vi "check_for_parse_errors.vi"(6 "just check details? (false: also raise labview error)":bool, 7 "optional file path (to include in parse error message)":path, 8 "error in (no error)":errorcluster, 11 "toml":string) -> (0 "error out":errorcluster, 1 "error details":string, 2 "error occurred?":bool)   [LabVIEW 2020, in "toml_edit.lvlib" / "Doc.lvclass"]
uses:
  Doc.lvclass
  <userlib>/_OpenG.lib/file/file.llb/Valid Path - Traditional__ogtk.vi
  toml_edit.lvlib
  <userlib>/_OpenG.lib/file/file.llb/openg_file.lvlib
  dragon_toml_64.dll
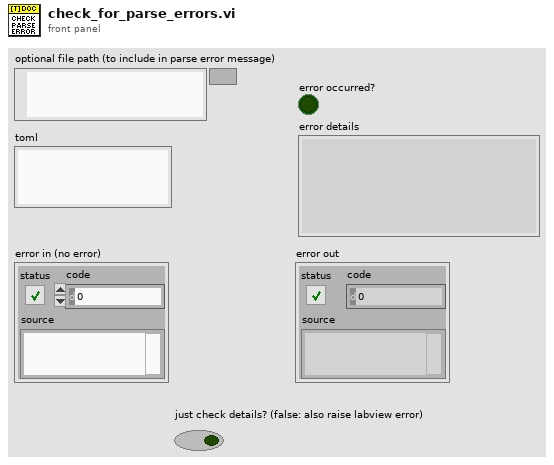
[diagram p1: front panel]
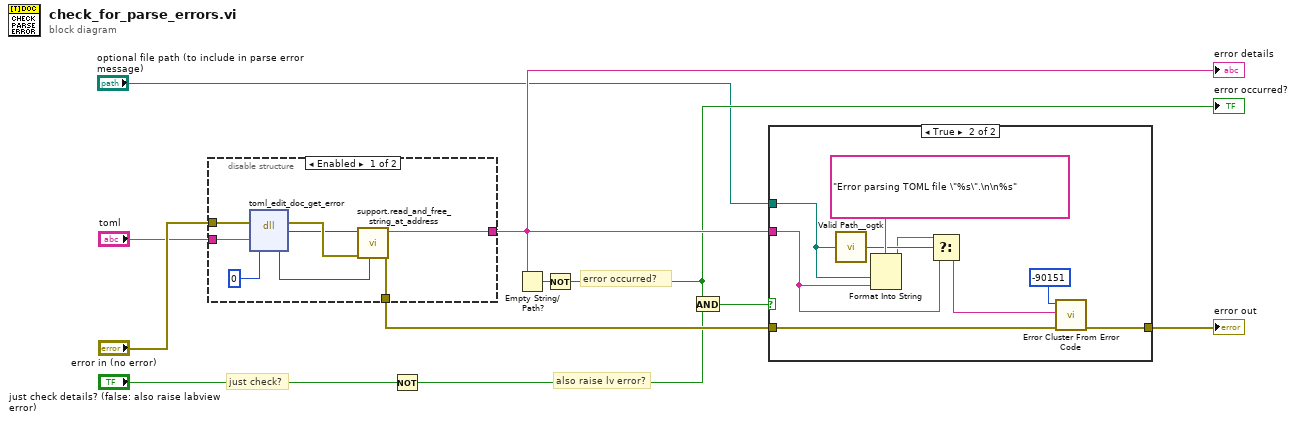
[diagram p0: block diagram]
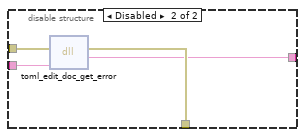
[diagram p2: hidden frame]
diagram:
  # "error occurred?"
  # "just check?"
  # "also raise lv error?"
  n1 = disable-structure shown="Enabled" {
    disable-tunnel: [w19 w21] -> w11
    disable-tunnel: [w18 w23] -> w8
    disable-tunnel: "error in (no error)" -> [w16 w22]
    disable-tunnel: "toml" -> [w14 w20]
    frame Enabled {
      n2 = dll-call lib="C:/projects/dragon-desktop/source/submodules/toml-edit-labview/lv_src/dragon_toml_*.*" fn="toml_edit_doc_get_error"(error in=w16, "toml_string"=w14, "string_length"=u32 0) -> (error out=w17:errorcluster, "error_string_ptr"=w15:u64, "string_length"=w13:u32)  [unwired: 3 in, 1 out]
      n3 = call "support.read_and_free_string_at_address.vi"("string_length"=w13, "error in (no error)"=w17, "string_ptr"=w15) -> ("error out"=w18:errorcluster, "string"=w19:string)  [unwired: 7 in]
    }
    frame Disabled {
      n4 = dll-call lib="C:/projects/dragon-desktop/source/submodules/toml-edit-labview/lv_src/dragon_toml_*.*" fn="toml_edit_doc_get_error"(error in=w22, "toml_string"=w20) -> (error out=w23:errorcluster, "error_string_ptr"=w21:string)  [unwired: 3 in, 1 out]
    }
  }
  "error details" <- w11
  n5 = Not(x="just check details? (false: also raise labview error)") -> (.not. x?=w2:bool)
  n6 = Empty String/Path?(string/path=w11) -> (empty?=w10:bool)
  n7 = Not(x=w10) -> (.not. x?=w5:bool)
  "error occurred?" <- w5
  n8 = And(x=w5, y=w2) -> (x .and. y?=w4:bool)
  n9 = case shown="True" w4 {
    tunnel: w8 -> [w24 w33]
    tunnel: [w24 w32] -> w9
    tunnel: w11 -> [_ w25]
    tunnel: "optional file path (to include in parse error message)" -> [_ w29]
    frame False {
    }
    frame True {
      n10 = call-poly <userlib>:"Valid Path__ogtk.vi"("path"=w29) -> ("valid"=w28:bool)
      n11 = Format Into String(format string="Error parsing TOML file \"%s\".\n\n%s", w29, w25) -> (resulting string=w27:string)  [unwired: 2 in, 1 out]
      n12 = Select(t=w27, s=w28, f=w25) -> (s? t:f=w26:string)
      n13 = call <vilib>:"Error Cluster From Error Code.vi"("error in (no error)"=w33, "error message (\"\")"=w26, "error code (0)"=-90151) -> ("error out"=w32:errorcluster)  [unwired: 6 in]
    }
  }
  "error out" <- w9
